vi "readFromXML.vi"(8 "error in (no error)":errorcluster, 10 "XML in":string="<DifftrackRADec>\n<dRA_ArcsPS>5.5</dRA_ArcsPS>\n<dDec_ArcsPS>10.2</dDec_ArcsPS>\n</DifftrackRADec>", 11 "DifftrackRADec in":refnum<class "DifftrackRADec.lvclass">) -> (0 "error out":errorcluster, 3 "DifftrackRADec out":refnum<class "DifftrackRADec.lvclass">)   [LabVIEW 2014, in "TCSDataDefinitions.lvlib" / "TCSCommand.lvlib" / "TargetConfiguration.lvlib" / "Target.lvlib" / "DifftrackRADec.lvclass"]
uses:
  DifftrackRADec.lvclass
  <userlib>/Common/UnitsAndXML/FlattenItemWithUnitToXML/FlattenAngularVelocityToXML/AngularVelocityUnit.ctl
  DifftrackRADec.lvclass/DifftrackRADec.ctl
  Difftrack.lvclass
  <userlib>/Common/UnitsAndXML/UnitsAndXML.lvlib
  <userlib>/Common/XML/XMLParser/XMLParser.lvclass
panel:
  out "dDec_ArcsPS":dbl[unit]=5.9147269095363384e-05
  out "dRA_ArcsPS":dbl[unit]=5.9147269095363384e-05
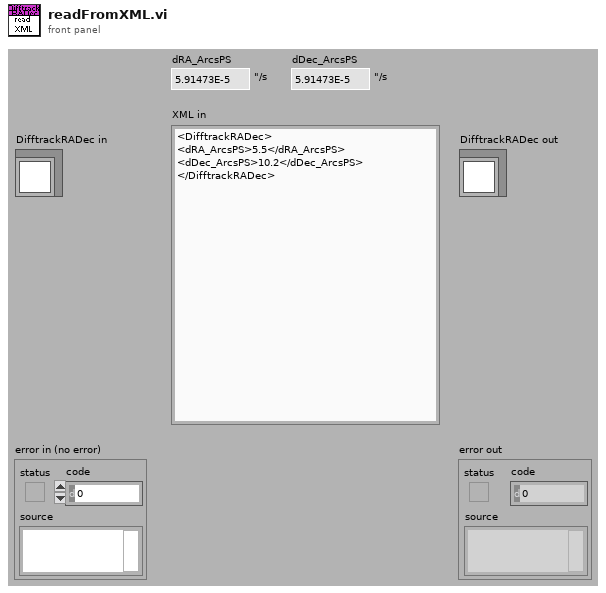
[diagram p1: front panel]
types:
  T1 = typedef "UnitsAndXML.lvlib/AngularVelocityUnit.ctl" = enum16{"\"/a", "deg/s", "\"/s"}
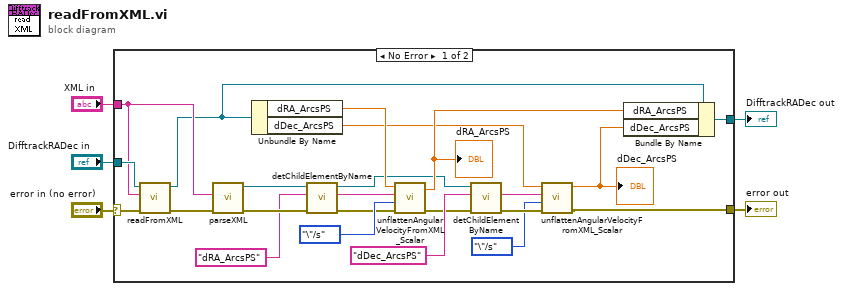
[diagram p0: block diagram]
diagram:
  n1 = case shown="No Error" "error in (no error)" {
    selector: "error in (no error)" -> [w23 w29]
    tunnel: [w8 w29] -> w5
    tunnel: [w18 w30] -> w4
    tunnel: "XML in" -> [w27 _]
    tunnel: "DifftrackRADec in" -> [w28 w30]
    frame No Error {
      n2 = call-parent "readFromXML.vi"("error in (no error)"=w23, "XML in"=w27, "Difftrack in"=w28) -> ("error out"=w22:errorcluster, "Difftrack out"=w19:refnum<class "DifftrackRADec.lvclass">)  [unwired: 7 in]
      n3 = call <userlib>:"parseXML.vi"("error in (no error)"=w22, "XMLString in"=w27) -> ("error out"=w26:errorcluster, "Element out"=w13:refnum<class "XMLParser.lvclass">)  [unwired: 8 in]
      n4 = Unbundle By Name(w19) -> ("dRA_ArcsPS"=w20:dbl[unit], "dDec_ArcsPS"=w7:dbl[unit])
      n5 = call <userlib>:"detChildElementByName.vi"("error in (no error)"=w26, "childName"="dRA_ArcsPS" ("ChildName"), "Element in"=w13) -> ("error out"=w14:errorcluster, "childXML"=w21:string, "Element out"=w12:refnum<class "XMLParser.lvclass">)  [unwired: 5 in, 1 out]
      n6 = call <userlib>:"unflattenAngularVelocityFromXML_Scalar.vi"("error in (no error)"=w14, "angularVelocityUnitInXML"=AngularVelocityUnit."\"/s", "xmlString"=w21, "angularVelocityForType"=w20) -> ("error out"=w15:errorcluster, "angularVelocity"=w17:dbl[unit])  [unwired: 6 in]
      "dRA_ArcsPS" <- w17
      n7 = call <userlib>:"detChildElementByName.vi"("error in (no error)"=w15, "childName"="dDec_ArcsPS" ("ChildName"), "Element in"=w12) -> ("error out"=w11:errorcluster, "childXML"=w9:string)  [unwired: 5 in, 2 out]
      n8 = call <userlib>:"unflattenAngularVelocityFromXML_Scalar.vi"("error in (no error)"=w11, "angularVelocityUnitInXML"=AngularVelocityUnit."\"/s", "xmlString"=w9, "angularVelocityForType"=w7) -> ("error out"=w8:errorcluster, "angularVelocity"=w6:dbl[unit])  [unwired: 6 in]
      "dDec_ArcsPS" <- w6
      n9 = Bundle By Name(cluster=w19, "dRA_ArcsPS"=w17, "dDec_ArcsPS"=w6) -> (w18:refnum<class "DifftrackRADec.lvclass">)
    }
    frame Error {
    }
  }
  "error out" <- w5
  "DifftrackRADec out" <- w4
